vi "EmsaInitializeQbus.vi"(8 "error in (no error)":errorcluster) -> (0 "error out":errorcluster, 3 "Qbus out":refnum<class "Qbus.lvclass">)   [LabVIEW 2017]
uses:
  <vilib>/addons/Qbus/Qbus.lvclass
  <vilib>/addons/BlinkProcess/BlinkProcess.lvlib
  <vilib>/addons/TimerProcess/TimerProcess.lvlib
  <vilib>/addons/InsightCM/Devices/Shared/Common/ServerComm/ServerComm.lvlib
  <vilib>/addons/InsightCM/Devices/Shared/Common/Trigger/Trigger.lvlib
  <vilib>/addons/TraceLogger/TraceLogger.lvlib
  <vilib>/addons/InsightCM/Devices/Shared/Common/Controller/Controller.lvlib
  <vilib>/addons/InsightCM/Devices/Shared/Common/DeviceHealth/DeviceHealth.lvlib
  <vilib>/addons/InsightCM/Devices/Shared/Common/FileManager/FileManager.lvlib
  <vilib>/addons/InsightCM/Devices/Shared/Emsa/EmsaAcquisition/EmsaAcquisition.lvlib
  <vilib>/addons/InsightCM/Devices/Shared/Emsa/EmsaAnalysis/EmsaAnalysis.lvlib
  <vilib>/addons/InsightCM/Devices/Shared/Emsa/EmsaDataFlowManager/EmsaDataFlowManager.lvlib
  <vilib>/addons/InsightCM/Devices/Shared/Emsa/EmsaAudio/EmsaAudio.lvlib
  <vilib>/addons/InsightCM/Devices/Shared/Common/OpState/OpState.lvlib
  <vilib>/addons/InsightCM/Devices/Shared/Common/TrendAlarm/TrendAlarm.lvlib
  <vilib>/addons/InsightCM/Devices/Shared/Emsa/EmsaFPGABifileManager/EmsaFPGABitfileManager.lvlib
  <vilib>/addons/InsightCM/Devices/Shared/Emsa/EmsaDataEventCreator/EmsaDataEventCreator.lvlib
  <vilib>/addons/InsightCM/Devices/Shared/Emsa/EmsaTestPanel/EmsaTestPanel.lvlib
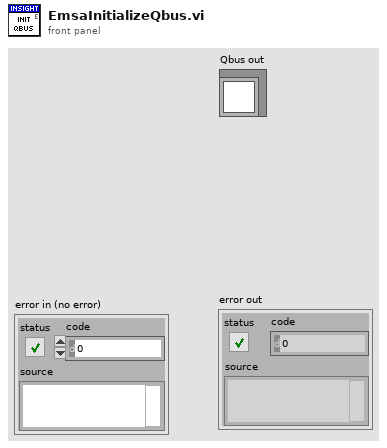
[diagram p1: front panel]
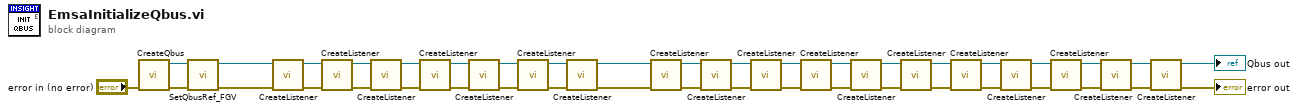
[diagram p0: block diagram]
diagram:
  n1 = call <vilib>:"CreateQbus.vi"("error in (no error)"="error in (no error)") -> ("error out"=w36:errorcluster, "Qbus"=w35:refnum<class "Qbus.lvclass">)  [unwired: 9 in]
  n2 = call <vilib>:"SetQbusRef_FGV.vi"("error in (no error)"=w36, "Qbus in"=w35) -> ("error out"=w9:errorcluster, "Qbus out"=w10:refnum<class "Qbus.lvclass">)  [unwired: 8 in]
  n3 = call <vilib>:"CreateListener.vi"("error in (no error)"=w9, "Qbus in"=w10) -> ("error out"=w19:errorcluster, "Qbus out"=w20:refnum<class "Qbus.lvclass">)  [unwired: 8 in]
  n4 = call <vilib>:"CreateListener.vi"("error in (no error)"=w19, "Qbus in"=w20) -> ("error out"=w17:errorcluster, "Qbus out"=w18:refnum<class "Qbus.lvclass">)  [unwired: 8 in]
  n5 = call <vilib>:"CreateListener.vi"("error in (no error)"=w17, "Qbus in"=w18) -> ("error out"=w28:errorcluster, "Qbus out"=w27:refnum<class "Qbus.lvclass">)  [unwired: 8 in]
  n6 = call <vilib>:"CreateListener.vi"("error in (no error)"=w28, "Qbus in"=w27) -> ("error out"=w30:errorcluster, "Qbus out"=w29:refnum<class "Qbus.lvclass">)  [unwired: 8 in]
  n7 = call <vilib>:"CreateListener.vi"("error in (no error)"=w30, "Qbus in"=w29) -> ("error out"=w15:errorcluster, "Qbus out"=w16:refnum<class "Qbus.lvclass">)  [unwired: 8 in]
  n8 = call <vilib>:"CreateListener.vi"("error in (no error)"=w15, "Qbus in"=w16) -> ("error out"=w11:errorcluster, "Qbus out"=w12:refnum<class "Qbus.lvclass">)  [unwired: 8 in]
  n9 = call <vilib>:"CreateListener.vi"("error in (no error)"=w11, "Qbus in"=w12) -> ("error out"=w4:errorcluster, "Qbus out"=w5:refnum<class "Qbus.lvclass">)  [unwired: 8 in]
  n10 = call <vilib>:"CreateListener.vi"("error in (no error)"=w4, "Qbus in"=w5) -> ("error out"=w3:errorcluster, "Qbus out"=w6:refnum<class "Qbus.lvclass">)  [unwired: 8 in]
  n11 = call <vilib>:"CreateListener.vi"("error in (no error)"=w3, "Qbus in"=w6) -> ("error out"=w8:errorcluster, "Qbus out"=w7:refnum<class "Qbus.lvclass">)  [unwired: 8 in]
  n12 = call <vilib>:"CreateListener.vi"("error in (no error)"=w8, "Qbus in"=w7) -> ("error out"=w13:errorcluster, "Qbus out"=w14:refnum<class "Qbus.lvclass">)  [unwired: 8 in]
  n13 = call <vilib>:"CreateListener.vi"("error in (no error)"=w13, "Qbus in"=w14) -> ("error out"=w24:errorcluster, "Qbus out"=w23:refnum<class "Qbus.lvclass">)  [unwired: 8 in]
  n14 = call <vilib>:"CreateListener.vi"("error in (no error)"=w24, "Qbus in"=w23) -> ("error out"=w21:errorcluster, "Qbus out"=w22:refnum<class "Qbus.lvclass">)  [unwired: 8 in]
  n15 = call <vilib>:"CreateListener.vi"("error in (no error)"=w21, "qbus in"=w22) -> ("error out"=w34:errorcluster, "qbus out"=w33:refnum<class "Qbus.lvclass">)  [unwired: 8 in]
  n16 = call <vilib>:"CreateListener.vi"("error in (no error)"=w34, "Qbus in"=w33) -> ("error out"=w26:errorcluster, "Qbus out"=w25:refnum<class "Qbus.lvclass">)  [unwired: 8 in]
  n17 = call <vilib>:"CreateListener.vi"("error in (no error)"=w26, "Qbus in"=w25) -> ("error out"=w2:errorcluster, "Qbus out"=w1:refnum<class "Qbus.lvclass">)  [unwired: 8 in]
  n18 = call <vilib>:"CreateListener.vi"("error in (no error)"=w2, "Qbus in"=w1) -> ("error out"=w31:errorcluster, "Qbus out"=w32:refnum<class "Qbus.lvclass">)  [unwired: 8 in]
  n19 = call <vilib>:"CreateListener.vi"("error in (no error)"=w31, "Qbus in"=w32) -> ("error out"=w40:errorcluster, "Qbus out"=w41:refnum<class "Qbus.lvclass">)  [unwired: 8 in]
  n20 = call <vilib>:"CreateListener.vi"("error in (no error)"=w40, "qbus in"=w41) -> ("error out"=→"error out":errorcluster, "qbus out"=→"Qbus out":refnum<class "Qbus.lvclass">)  [unwired: 8 in]
